vi "AppendPadNodes.vi"(8 "Error In":errorcluster, 9 "Input":T1, 10 "Input Node In":refnum<k20>, 11 "DOM Document":refnum<k20>) -> (0 "Error Out":errorcluster, 3 "Input Node Out":refnum<k20>)   [LabVIEW 2012, in "Virtual-PGA.lvlib"]
uses:
  Virtual-PGA.lvlib
  Public/Controls/Input.ctl
  <resource>/objmgr/DOMUserDefRef.rc
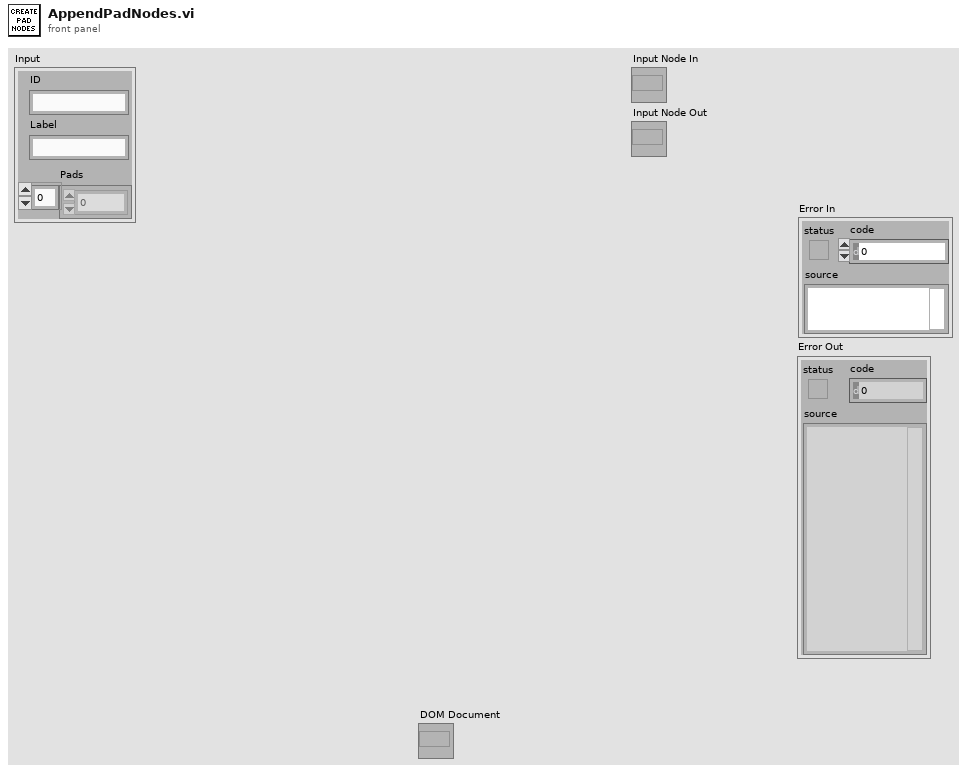
[diagram p1: front panel]
types:
  T1 = typedef "Virtual-PGA.lvlib/Input.ctl" = cluster{"ID":string, "Label":string, "Pads":u32[]}
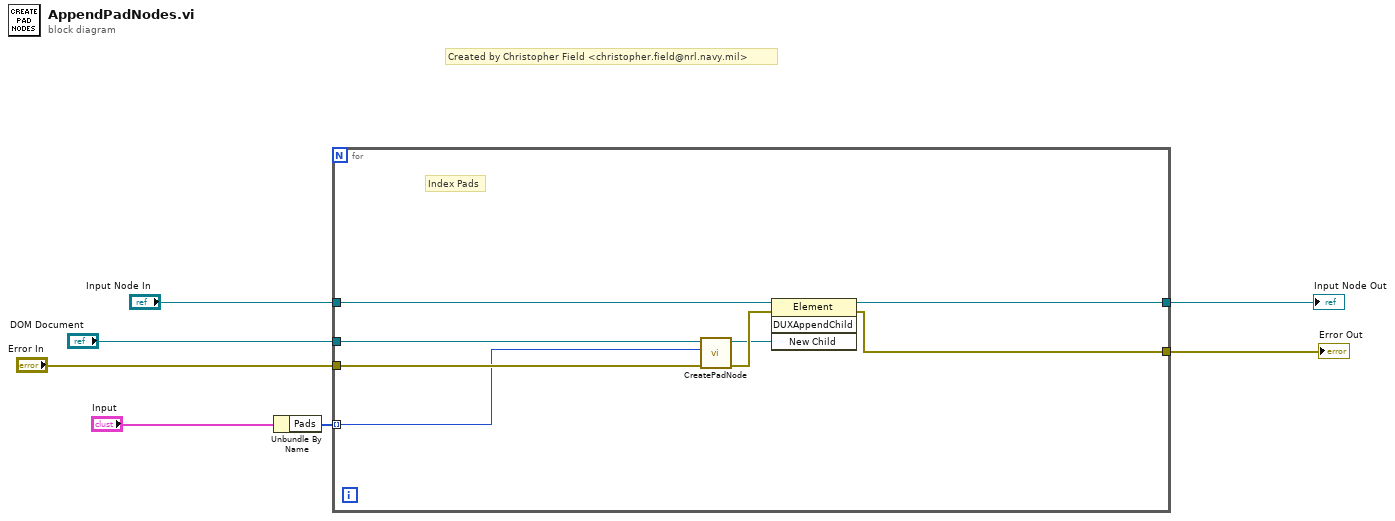
[diagram p0: block diagram]
diagram:
  # "Created by Christopher Field <christopher.field@nrl.navy.mil>"
  n1 = Unbundle By Name("Input") -> ("Pads"=w1:u32[])
  n2 = for {
    tunnel: "DOM Document" -> [w15]
    tunnel: "Error In" -> [w14]
    tunnel: [w13] -> w6
    tunnel: [w12] -> w5
    tunnel: "Input Node In" -> [w11]
    tunnel: w1 -> [w8] mode=indexing
    # "Index Pads"
    n3 = call "CreatePadNode.vi"("Error In"=w14, "Pad Number"=w8, "DOM Document"=w15) -> ("Error Out"=w10:errorcluster, "Pad Element"=w9:refnum<k20>)  [unwired: 7 in]
    n4 = invoke class="Element" method="DUXAppendChild"(reference=w11, error in=w10, "New Child"=w9) -> (reference out=w13:refnum<k20>, error out=w12:errorcluster)  [unwired: 1 in, 2 out]
  }
  "Error Out" <- w5
  "Input Node Out" <- w6
